vi "Teleop.vi"(10 "Match Info":T1={"Autonomous Elapsed Seconds"=0.0, "TeleOp Elapsed Seconds"=0.0, "Disabled Elapsed Seconds"=0.0, "Visited Autonomous"=FALSE, "Visited TeleOp"=FALSE, "Visited Disabled"=FALSE, "Autonomous Settings"={"Autonomous Style"=enum."Independent", "VI Refnum"=refnum}}, 11 "Call Context":T2=enum."Execute") -> ()   [LabVIEW 2018]
doc: "This VI is called for each TeleOp packet received from the DS where the robot is not disabled. It is often used to read from the joysticks and update I/O or to update setpoints for timed control loops. It should complete and return within 20 milliseconds or it may miss DS packets."
uses:
  <vilib>/Rock Robotics/Network Tables/NT Write Numeric Array.vi
  <vilib>/Rock Robotics/Network Tables/NT Read Boolean.vi
  <vilib>/Rock Robotics/Network Tables/NT Write Boolean Array.vi
  Globals.vi
  <vilib>/Rock Robotics/WPI/Solenoid/WPI_SolenoidValue.ctl
  <vilib>/Rock Robotics/WPI/Solenoid/WPI_SolenoidSetEnum.vi
  <vilib>/Rock Robotics/Network Tables/NT Write Boolean.vi
  <vilib>/Rock Robotics/Network Tables/NT Read Number.vi
  <vilib>/Rock Robotics/WPI/ThirdParty/Phoenix-LabVIEW/Motor Controller/Controls/CTRE_Phoenix_MotorControl_ControlMode.ctl
  Robot Global Data.vi
  <vilib>/Rock Robotics/WPI/DriverStation/WPI_DriverStationMatch Info.ctl
  <vilib>/Rock Robotics/WPI/DriverStation/WPI_DriverStationDerivedRobotMode.ctl
panel:
  out "Drive Mode":bool
  in  "Mode":string(combo)="Driving"
  out "Drive Type":bool
  out "Sample Slider 0":dbl(slide) scale=0.0..5.0
  out "Sample Boolean 1":bool
  out "Sample Boolean 0":bool
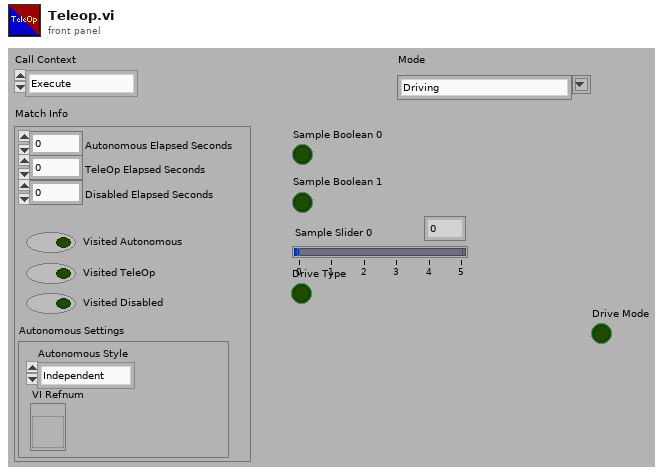
[diagram p1: front panel]
types:
  T1 = typedef "WPI_DriverStationMatch Info.ctl" = cluster{"Autonomous Elapsed Seconds":dbl, "TeleOp Elapsed Seconds":dbl, "Disabled Elapsed Seconds":dbl, "Visited Autonomous":bool, "Visited TeleOp":bool, "Visited Disabled":bool, "Autonomous Settings":cluster{"Autonomous Style":enum16{"Iterative", "Independent"}, "VI Refnum":refnum<vi>}}
  T2 = typedef "WPI_DriverStationDerivedRobotMode.ctl" = enum16{"Init", "Execute", "Stop"}
  T3 = typedef "WPI_RobotDriveDevRef.ctl" = cluster{"DevStatus":errorcluster, "Motors[]":T4[], "Square Inputs":bool, "Max Output":dbl}
  T4 = typedef "WPI_MotorControlDeviceRef.ctl" = cluster{"DeviceStatus":errorcluster, "Type":T5, "PWM":cluster{"PWM Channel":T6, "DeadBand":T7}, "CAN":cluster{"Device Number":u8, "SetOutput VI Ref":variant, "GetOutput VI Ref":variant, "Enable VI Ref":variant, "Disable VI Ref":variant, "Data":variant}, "Invert":bool, "DIO PWM":cluster{"PWM \"Enable\" Channel":T6, "DIOChannel":T8, "PWM Rate":dbl}}
  T5 = typedef "WPI_MotorControlType.ctl" = enum16{"PWM", "CAN", "DIO PWM"}
  T6 = typedef "FPGA_DIOPWMChannel.ctl" = enum8{"PWM 0", "PWM 1", "PWM 2", "PWM 3", "PWM 4", "PWM 5", "PWM 6", "PWM 7", "PWM 8", "PWM 9", "PWM MXP 0", "PWM MXP 1", "PWM MXP 2", "PWM MXP 3", "PWM MXP 4", "PWM MXP 5", "PWM MXP 6", "PWM MXP 7", "PWM MXP 8", "PWM MXP 9", "Invalid"}
  T7 = typedef "WPI_PWMDeadband.ctl" = cluster{"Name":string, "maxPositivePwm":i32, "minPositivePwm":i32, "centerPwm":i32, "maxNegativePwm":i32, "minNegativePwm":i32, "angularRange":u16}
  T8 = typedef "FPGA_DIOChannel.ctl" = enum8{"DIO 0", "DIO 1", "DIO 2", "DIO 3", "DIO 4", "DIO 5", "DIO 6", "DIO 7", "DIO 8", "DIO 9", "DIO MXP 0", "DIO MXP 1", "DIO MXP 2", "DIO MXP 3", "DIO MXP 4", "DIO MXP 5", "DIO MXP 6", "DIO MXP 7", "DIO MXP 8", "DIO MXP 9", "DIO MXP 10", "DIO MXP 11", "DIO MXP 12", "DIO MXP 13", "DIO MXP 14", "DIO MXP 15", "SPI Port CS1", "SPI Port CS2", "SPI Port CS3", "SPI Port MISO", "SPI Port MOSI", "Invalid"}
  T9 = typedef "WPI_JoystickDevRef.ctl" = cluster{"Device":T10}
  T10 = typedef "WPI_JoystickDeviceEnum.ctl" = enum16{"USB 0", "USB 1", "USB 2", "USB 3", "USB 4", "USB 5"}
  T11 = typedef "CTRE_Phoenix_MotorControl_ControlMode.ctl" = u16
  T12 = typedef "WPI_SolenoidValue.ctl" = enum16{"Off", "On", "Forward", "Reverse"}
  T13 = typedef "WPI_SolenoidDevRef.ctl" = cluster{"DevStatus":errorcluster, "Pneumatics Control Module":u8, "Forward Solenoid Channel":T14, "Reverse Solenoid Channel":T14}
  T14 = typedef "WPI_SolenoidChannel.ctl" = enum8{"Solenoid 0", "Solenoid 1", "Solenoid 2", "Solenoid 3", "Solenoid 4", "Solenoid 5", "Solenoid 6", "Solenoid 7", "Invalid"}
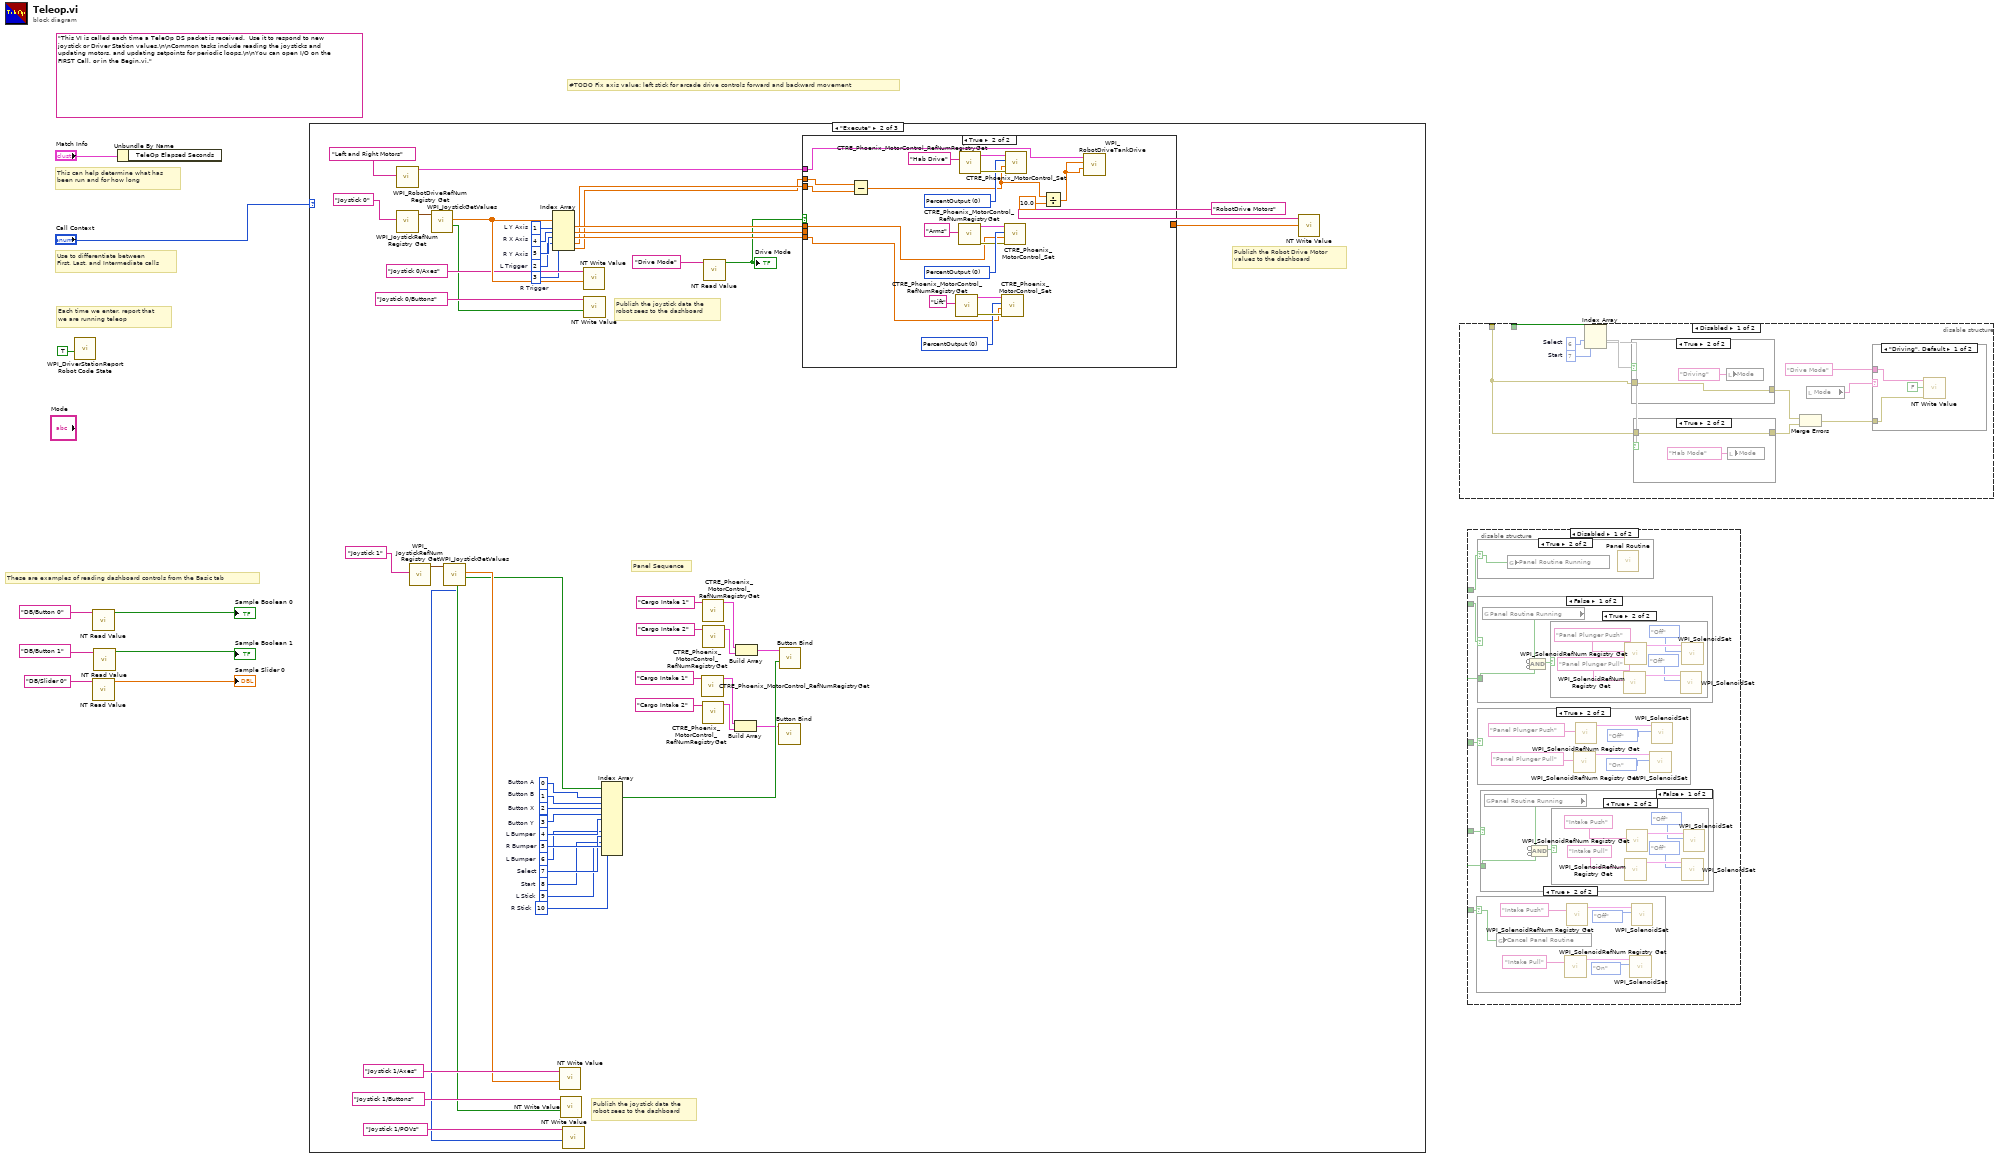
[diagram p0: block diagram]
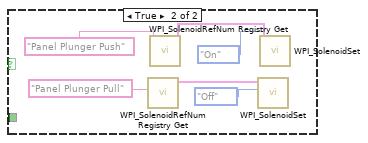
[diagram p4: hidden frame]
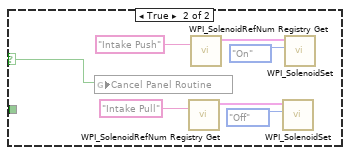
[diagram p7: hidden frame]
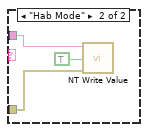
[diagram p10: hidden frame]
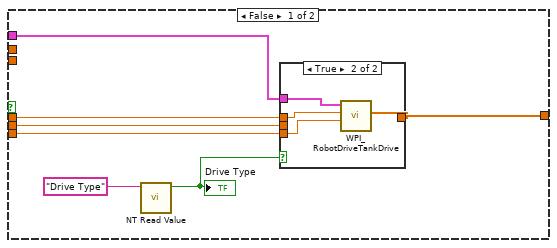
[diagram p15: hidden frame]
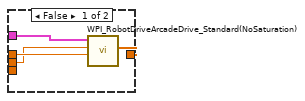
[diagram p16: hidden frame]
diagram:
  (unwired) "This VI is called each time a TeleOp DS packet is received.  Use it to respond to new joystick or Driver Station values.\n\nCommon tasks include reading the joysticks and updating motors, and updating setpoints for periodic loops.\n\nYou can open I/O on the FIRST Call, or in the Begin.vi."
  # "#TODO Fix axis value: left stick for arcade drive controls forward and backward movement"
  # "These are examples of reading dashboard controls from the Basic tab"
  # "Each time we enter, report that\nwe are running teleop"
  # "Use to differentiate between\nFirst, Last, and Intermediate calls"
  # "This can help determine what has\nbeen run and for how long"
  n1 = call <vilib>:"WPI_DriverStationReport Robot Code State.vi"("TeleOp"=TRUE ("Autonomous")) -> ()  [unwired: 10 in, 1 out]
  n2 = call-poly <vilib>:"NT Read Value.vi"("Name"="DB/Button 0" ("refnum name")) -> ("Boolean"=→"Sample Boolean 0":bool)  [unwired: 9 in, 1 out]
  n3 = call-poly <vilib>:"NT Read Value.vi"("Name"="DB/Slider 0" ("refnum name")) -> ("Numeric"=→"Sample Slider 0":dbl)  [unwired: 9 in, 1 out]
  n4 = call-poly <vilib>:"NT Read Value.vi"("Name"="DB/Button 1" ("refnum name")) -> ("Boolean"=→"Sample Boolean 1":bool)  [unwired: 9 in, 1 out]
  n5 = Unbundle By Name("Match Info") -> ()  [unwired: 1 out]
  n6 = case shown="\"Execute\"" "Call Context" {
    frame "Init", Default {
    }
    frame "Execute" {
      w10 = 10  # R Stick
      w11 = 9  # L Stick
      w12 = 8  # Start
      w13 = 7  # Select
      w14 = 6  # L Bumper
      w15 = 5  # R Bumper
      w29 = 3  # R Trigger
      w30 = 2  # L Trigger
      w34 = 4  # L Bumper
      w46 = 3  # Button Y
      w43 = 1  # Button B
      w45 = 0  # Button A
      w44 = 2  # Button X
      w51 = 4  # R X Axis
      w52 = 1  # L Y Axis
      w50 = 5  # R Y Axis
      # "Publish the joystick data the\nrobot sees to the dashboard"
      # "Panel Sequence"
      # "Publish the Robot Drive Motor\nvalues to the dashboard"
      # "Publish the joystick data the\nrobot sees to the dashboard"
      n7 = call <vilib>:"WPI_RobotDriveRefNum Registry Get.vi"("refnum name"="Left and Right Motors") -> ("RobotDriveDevRef"=w55:T3)  [unwired: 1 in, 9 out]
      n8 = call <vilib>:"WPI_JoystickRefNum Registry Get.vi"("refnum name"="Joystick 0") -> ("JoystickDevRef"=w60:T9)  [unwired: 1 in, 9 out]
      n9 = call <vilib>:"WPI_JoystickRefNum Registry Get.vi"("refnum name"="Joystick 1") -> ("JoystickDevRef"=w41:T9)  [unwired: 1 in, 9 out]
      n10 = call <vilib>:"WPI_JoystickGetValues.vi"("JoystickDevRef"=w60) -> ("Buttons"=w33:bool[], "Axes"=w61:dbl[])  [unwired: 6 in, 3 out]
      n11 = call <vilib>:"WPI_JoystickGetValues.vi"("JoystickDevRef"=w41) -> ("Buttons"=w37:bool[], "Axes"=w38:dbl[], "POVs"=w35:i16[])  [unwired: 6 in, 2 out]
      n12 = Index Array(array=w61, index #1=w52, index #2=w51, index #3=w50, index #4=w30, index #5=w29) -> (element #1=w47:dbl, element #2=w48:dbl, element #3=w49:dbl, element #4=w28:dbl, element #5=w27:dbl)
      n13 = call-poly <vilib>:"NT Write Value.vi"("Numeric Array"=w38, "Name"="Joystick 1/Axes") -> ()  [unwired: 9 in, 1 out]
      n14 = call-poly <vilib>:"NT Write Value.vi"("Boolean Array"=w37, "Name"="Joystick 1/Buttons") -> ()  [unwired: 9 in, 1 out]
      n15 = call-poly <vilib>:"NT Write Value.vi"("Numeric Array"=w35, "Name"="Joystick 1/POVs") -> ()  [unwired: 9 in, 1 out]
      n16 = call-poly <vilib>:"NT Write Value.vi"("Numeric Array"=w61, "Name"="Joystick 0/Axes") -> ()  [unwired: 9 in, 1 out]
      n17 = call-poly <vilib>:"NT Write Value.vi"("Boolean Array"=w33, "Name"="Joystick 0/Buttons") -> ()  [unwired: 9 in, 1 out]
      n18 = Index Array(array=w37, index #1=w45, index #2=w43, index #3=w44, index #4=w46, index #5=w34, index #6=w15, index #7=w14, index #8=w13, index #9=w12, index #10=w11, index #11=w10) -> (element #1=w21:bool)  [unwired: 10 out]
      n19 = call <vilib>:"CTRE_Phoenix_MotorControl_RefNumRegistryGet.vi"("refnum name"="Cargo Intake 1") -> ("PhoenixMotorControlDevRef"=w18:T4)  [unwired: 9 in, 1 out]
      n20 = call <vilib>:"CTRE_Phoenix_MotorControl_RefNumRegistryGet.vi"("refnum name"="Cargo Intake 1") -> ("PhoenixMotorControlDevRef"=w24:T4)  [unwired: 9 in, 1 out]
      n21 = call <vilib>:"CTRE_Phoenix_MotorControl_RefNumRegistryGet.vi"("refnum name"="Cargo Intake 2") -> ("PhoenixMotorControlDevRef"=w19:T4)  [unwired: 9 in, 1 out]
      n22 = call <vilib>:"CTRE_Phoenix_MotorControl_RefNumRegistryGet.vi"("refnum name"="Cargo Intake 2") -> ("PhoenixMotorControlDevRef"=w23:T4)  [unwired: 9 in, 1 out]
      n23 = call-poly <vilib>:"NT Read Value.vi"("Name"="Drive Mode" ("refnum name")) -> ("Boolean"=w31:bool)  [unwired: 9 in, 1 out]
      "Drive Mode" <- w31
      n24 = Build Array(w18, w19) -> (w20:T4[])
      n25 = Build Array(w24, w23) -> (w22:T4[])
      n26 = call "Button Bind.vi"("Motor Controllers"=w20) -> ()  [unwired: 11 in]
      n27 = call "Button Bind.vi"("Button Input"=w21, "Motor Controllers"=w22) -> ()  [unwired: 10 in]
      n28 = case shown="True" w31 {
        tunnel: w55 -> [w68 w80]
        tunnel: [w67 _] -> w54
        tunnel: w49 -> [w64 w83]
        tunnel: w48 -> [w63 _]
        tunnel: w47 -> [w62 w84]
        tunnel: w28 -> [_ w81]
        tunnel: w27 -> [_ w82]
        frame False {
          n29 = call-poly <vilib>:"NT Read Value.vi"("Name"="Drive Type" ("refnum name")) -> ("Boolean"=w65:bool)  [unwired: 9 in, 1 out]
          "Drive Type" <- w65
          n30 = case shown="True" w65 {
            tunnel: w68 -> [w71 w76]
            tunnel: [w72 w75] -> w67
            tunnel: w64 -> [_ w73]
            tunnel: w63 -> [w69 _]
            tunnel: w62 -> [w70 w74]
            frame False {
              n31 = call <vilib>:"WPI_RobotDriveArcadeDrive_Standard(NoSaturation).vi"("Y axis value"=w70, "X axis value"=w69, "RobotDriveDevRef"=w71) -> ("Motor Values"=w72:dbl[])  [unwired: 1 in, 7 out]
            }
            frame True {
              n32 = call <vilib>:"WPI_RobotDriveTankDrive.vi"("Right axis value"=w73, "Left axis value"=w74, "RobotDriveDevRef"=w76) -> ("Motor Values"=w75:dbl[])  [unwired: 6 in, 2 out]
            }
          }
        }
        frame True {
          w85 = T11 0 items=["PercentOutput"=0, "Position"=1, "Velocity"=2, "Current"=3, "Follower"=5, "MotionProfile"=6, "MotionMagic"=7, "MotionProfileArc"=10, "Disabled"=15] ("Control Mode")
          w92 = T11 0 items=["PercentOutput"=0, "Position"=1, "Velocity"=2, "Current"=3, "Follower"=5, "MotionProfile"=6, "MotionMagic"=7, "MotionProfileArc"=10, "Disabled"=15] ("Control Mode")
          w93 = T11 0 items=["PercentOutput"=0, "Position"=1, "Velocity"=2, "Current"=3, "Follower"=5, "MotionProfile"=6, "MotionMagic"=7, "MotionProfileArc"=10, "Disabled"=15] ("Control Mode")
          n33 = Subtract(x=w82, y=w81) -> (x-y=w78:dbl)
          n34 = call <vilib>:"CTRE_Phoenix_MotorControl_RefNumRegistryGet.vi"("refnum name"="Lift") -> ("error out"=w86:errorcluster, "PhoenixMotorControlDevRef"=w87:T4)  [unwired: 9 in]
          n35 = call <vilib>:"CTRE_Phoenix_MotorControl_RefNumRegistryGet.vi"("refnum name"="Arms") -> ("error out"=w91:errorcluster, "PhoenixMotorControlDevRef"=w90:T4)  [unwired: 9 in]
          n36 = call <vilib>:"CTRE_Phoenix_MotorControl_RefNumRegistryGet.vi"("refnum name"="Hab Drive") -> ("error out"=w94:errorcluster, "PhoenixMotorControlDevRef"=w95:T4)  [unwired: 9 in]
          n37 = call <vilib>:"CTRE_Phoenix_MotorControl_Set.vi"("error in (no error)"=w86, "Output"=w83, "Control Mode"=w85, "PhoenixMotorControlDevRef"=w87) -> ()  [unwired: 6 in, 2 out]
          n38 = call <vilib>:"CTRE_Phoenix_MotorControl_Set.vi"("error in (no error)"=w91, "Output"=w84, "Control Mode"=w92, "PhoenixMotorControlDevRef"=w90) -> ()  [unwired: 6 in, 2 out]
          n39 = call <vilib>:"CTRE_Phoenix_MotorControl_Set.vi"("error in (no error)"=w94, "Output"=w78, "Control Mode"=w93, "PhoenixMotorControlDevRef"=w95) -> ()  [unwired: 6 in, 2 out]
          n40 = Divide(x=w78, y=10.0) -> (x/y=w77:dbl)
          n41 = call <vilib>:"WPI_RobotDriveTankDrive.vi"("Right axis value"=w77, "Left axis value"=w77, "RobotDriveDevRef"=w80) -> ()  [unwired: 6 in, 3 out]
        }
      }
      n42 = call-poly <vilib>:"NT Write Value.vi"("Numeric Array"=w54, "Name"="RobotDrive Motors") -> ()  [unwired: 9 in, 1 out]
    }
    frame "Stop" {
    }
  }
  n43 = disable-structure shown="Disabled" {
    disable-tunnel: _ -> [w107 _]
    disable-tunnel: _ -> [w102 _]
    frame Disabled {
      w105 = 7  # Start
      w106 = 6  # Select
      n44 = Index Array(array=w107, index #1=w106, index #2=w105) -> (element #1=w104, element #2=w103)
      n45 = case shown="True" w104 {
        tunnel: w102 -> [_ w116]
        tunnel: [_ w116] -> w100
        frame False {
        }
        frame True {
          n46 = local write "Mode"("Driving" ("Mode")) -> ()
        }
      }
      n47 = case shown="True" w103 {
        tunnel: w102 -> [_ w114]
        tunnel: [_ w114] -> w101
        frame False {
        }
        frame True {
          n48 = local write "Mode"("Hab Mode" ("Mode")) -> ()
        }
      }
      n49 = Merge Errors(w100, w101) -> (w99:errorcluster)
      n50 = local read "Mode"() -> (w97:string)
      n51 = case shown="\"Driving\", Default" w97 {
        tunnel: w99 -> [w110 w113]
        tunnel: "Drive Mode" ("refnum name") -> [w109 w112]
        frame "Driving", Default {
          n52 = call-poly <vilib>:"NT Write Value.vi"("error in"=w110, "Boolean"=FALSE, "Name"=w109) -> ()  [unwired: 8 in, 1 out]
        }
        frame "Hab Mode" {
          n53 = call-poly <vilib>:"NT Write Value.vi"("error in"=w113, "Boolean"=TRUE, "Name"=w112) -> ()  [unwired: 8 in, 1 out]
        }
      }
    }
    frame Enabled {
    }
  }
  n54 = disable-structure shown="Disabled" {
    disable-tunnel: _ -> [w122 _]
    disable-tunnel: _ -> [w121 _]
    disable-tunnel: _ -> [w120 _]
    disable-tunnel: _ -> [w119 _]
    disable-tunnel: _ -> [w118 _]
    frame Disabled {
      n55 = case shown="True" w118 {
        selector: w118 -> [_ w144]
        frame False {
        }
        frame True {
          n56 = global write "Robot Global Data.vi" "Cancel Panel Routine"(w144) -> ()
          n57 = call <vilib>:"WPI_SolenoidRefNum Registry Get.vi"("refnum name"="Intake Pull") -> ("SolenoidDevRef"=w147:T13)  [unwired: 9 in, 1 out]
          n58 = call <vilib>:"WPI_SolenoidRefNum Registry Get.vi"("refnum name"="Intake Push") -> ("SolenoidDevRef"=w148:T13)  [unwired: 9 in, 1 out]
          n59 = call-poly <vilib>:"WPI_SolenoidSet.vi"("Value"=WPI_SolenoidValue."On", "SolenoidDevRef"=w147) -> ()  [unwired: 1 in, 9 out]
          n60 = call-poly <vilib>:"WPI_SolenoidSet.vi"("Value"=WPI_SolenoidValue."Off", "SolenoidDevRef"=w148) -> ()  [unwired: 1 in, 9 out]
        }
      }
      n61 = case shown="True" w122 {
        selector: w122 -> [_ w167]
        frame False {
        }
        frame True {
          n62 = global write "Globals.vi" "Panel Routine Running"(w167) -> ()
          n63 = call "Panel Routine.vi"() -> ()  [unwired: 12 in]
        }
      }
      n64 = case shown="False" w120 {
        tunnel: w119 -> [w129 _]
        frame False {
          n65 = global read "Globals.vi" "Panel Routine Running"() -> (w130:bool)
          n66 = Compound Arithmetic op=AND(invert w130, invert w129) -> (w131:bool)
          n67 = case shown="True" w131 {
            frame False {
            }
            frame True {
              n68 = call <vilib>:"WPI_SolenoidRefNum Registry Get.vi"("refnum name"="Panel Plunger Pull") -> ("SolenoidDevRef"=w136:T13)  [unwired: 9 in, 1 out]
              n69 = call <vilib>:"WPI_SolenoidRefNum Registry Get.vi"("refnum name"="Panel Plunger Push") -> ("SolenoidDevRef"=w137:T13)  [unwired: 9 in, 1 out]
              n70 = call-poly <vilib>:"WPI_SolenoidSet.vi"("Value"=WPI_SolenoidValue."Off", "SolenoidDevRef"=w136) -> ()  [unwired: 1 in, 9 out]
              n71 = call-poly <vilib>:"WPI_SolenoidSet.vi"("Value"=WPI_SolenoidValue."Off", "SolenoidDevRef"=w137) -> ()  [unwired: 1 in, 9 out]
            }
          }
        }
        frame True {
          n72 = call <vilib>:"WPI_SolenoidRefNum Registry Get.vi"("refnum name"="Panel Plunger Pull") -> ("SolenoidDevRef"=w138:T13)  [unwired: 9 in, 1 out]
          n73 = call <vilib>:"WPI_SolenoidRefNum Registry Get.vi"("refnum name"="Panel Plunger Push") -> ("SolenoidDevRef"=w143:T13)  [unwired: 9 in, 1 out]
          n74 = call-poly <vilib>:"WPI_SolenoidSet.vi"("Value"=WPI_SolenoidValue."Off", "SolenoidDevRef"=w138) -> ()  [unwired: 1 in, 9 out]
          n75 = call-poly <vilib>:"WPI_SolenoidSet.vi"("Value"=WPI_SolenoidValue."On", "SolenoidDevRef"=w143) -> ()  [unwired: 1 in, 9 out]
        }
      }
      n76 = case shown="True" w119 {
        frame False {
        }
        frame True {
          n77 = call <vilib>:"WPI_SolenoidRefNum Registry Get.vi"("refnum name"="Panel Plunger Pull") -> ("SolenoidDevRef"=w123:T13)  [unwired: 9 in, 1 out]
          n78 = call <vilib>:"WPI_SolenoidRefNum Registry Get.vi"("refnum name"="Panel Plunger Push") -> ("SolenoidDevRef"=w128:T13)  [unwired: 9 in, 1 out]
          n79 = call-poly <vilib>:"WPI_SolenoidSet.vi"("Value"=WPI_SolenoidValue."On", "SolenoidDevRef"=w123) -> ()  [unwired: 1 in, 9 out]
          n80 = call-poly <vilib>:"WPI_SolenoidSet.vi"("Value"=WPI_SolenoidValue."Off", "SolenoidDevRef"=w128) -> ()  [unwired: 1 in, 9 out]
        }
      }
      n81 = case shown="False" w121 {
        selector: w121 -> [_ w160]
        tunnel: w118 -> [w151 _]
        frame False {
          n82 = global read "Robot Global Data.vi" "Panel Routine Running"() -> (w152:bool)
          n83 = Compound Arithmetic op=AND(invert w152, invert w151) -> (w153:bool)
          n84 = case shown="True" w153 {
            frame False {
            }
            frame True {
              n85 = call <vilib>:"WPI_SolenoidRefNum Registry Get.vi"("refnum name"="Intake Pull") -> ("SolenoidDevRef"=w158:T13)  [unwired: 9 in, 1 out]
              n86 = call <vilib>:"WPI_SolenoidRefNum Registry Get.vi"("refnum name"="Intake Push") -> ("SolenoidDevRef"=w159:T13)  [unwired: 9 in, 1 out]
              n87 = call-poly <vilib>:"WPI_SolenoidSet.vi"("Value"=WPI_SolenoidValue."Off", "SolenoidDevRef"=w158) -> ()  [unwired: 1 in, 9 out]
              n88 = call-poly <vilib>:"WPI_SolenoidSet.vi"("Value"=WPI_SolenoidValue."Off", "SolenoidDevRef"=w159) -> ()  [unwired: 1 in, 9 out]
            }
          }
        }
        frame True {
          n89 = global write "Globals.vi" "Cancel Panel Routine"(w160) -> ()
          n90 = call <vilib>:"WPI_SolenoidRefNum Registry Get.vi"("refnum name"="Intake Pull") -> ("SolenoidDevRef"=w163:T13)  [unwired: 9 in, 1 out]
          n91 = call <vilib>:"WPI_SolenoidRefNum Registry Get.vi"("refnum name"="Intake Push") -> ("SolenoidDevRef"=w164:T13)  [unwired: 9 in, 1 out]
          n92 = call-poly <vilib>:"WPI_SolenoidSet.vi"("Value"=WPI_SolenoidValue."Off", "SolenoidDevRef"=w163) -> ()  [unwired: 1 in, 9 out]
          n93 = call-poly <vilib>:"WPI_SolenoidSet.vi"("Value"=WPI_SolenoidValue."On", "SolenoidDevRef"=w164) -> ()  [unwired: 1 in, 9 out]
        }
      }
    }
    frame Enabled {
    }
  }
